vi "Time.vi"(8 "error in (no error)":errorcluster, 10 "Control In":T1={"I-O.lvclass"=refnum, "Gantry"=refnum, "Dispenser"="COM1"}, 11 "Sensor Dispense in":refnum<class "Sensor Dispense.lvclass">) -> (0 "error out":errorcluster, 1 "Timing Data":i32[](array[numeric]), 2 "Control Out":T1={"I-O.lvclass"=refnum, "Gantry"=refnum, "Dispenser"="COM1"}, 3 "Sensor Dispense out":refnum<class "Sensor Dispense.lvclass">)   [LabVIEW 2018, in "Sensor Dispense.lvclass"]
uses:
  Projects/Sensor Dispense.lvclass
  C:/Users/HEP/Documents/GitHub/New folder/C/Users/HEP/Documents/GitHub/UCSB-Gantry-HEP-2018/Classes/Routine/Dispense/Dispense.lvclass
  Controller/Controllers.ctl
  Controller/I-O/I-O.lvclass
  C:/Program Files (x86)/Aerotech/A3200/LabVIEW/2010/Bin/Aerotech.A3200.dll
  Program Files (x86)/Aerotech/A3200/LabVIEW/2010/Bin/Aerotech.A3200.dll
  Projects/Sensor Dispense.lvclass/Sensor Dispense.ctl
  Controller/Motion/Motion.lvclass
  Controller/Motion/A3200/A3200.lvclass
  Controller/Controller.lvclass
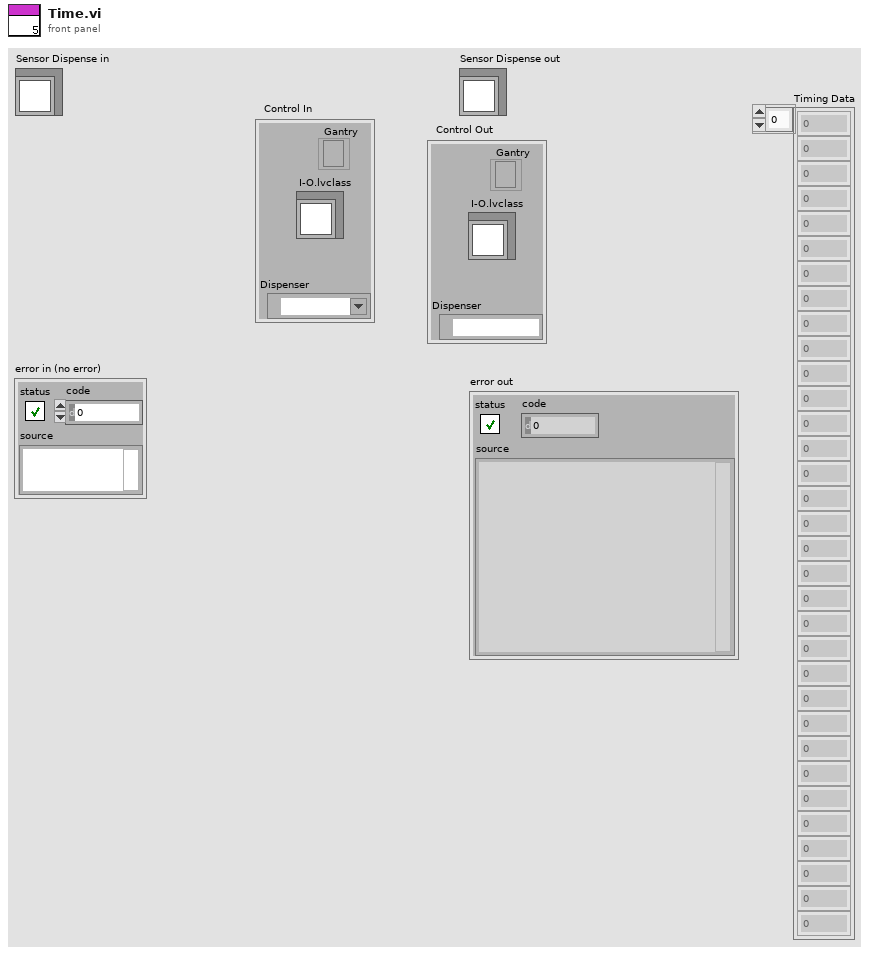
[diagram p1: front panel]
types:
  T1 = typedef "Controller.lvclass/Controllers.ctl" = cluster{"I-O.lvclass":refnum<class "I-O.lvclass">, "Gantry":refnum<k24>, "Dispenser":refnum<visa-resource-name>}
  T2 = cluster{"Endpoints":dbl[][], "Center":dbl[], "CW/CCW":dbl, "Dispense Type":enum16{"N-gon", "Square", "Arc", "Dot", "Line", "Circle"}}[]
  T3 = enum16{"N-gon", "Square", "Arc", "Dot", "Line", "Circle"}
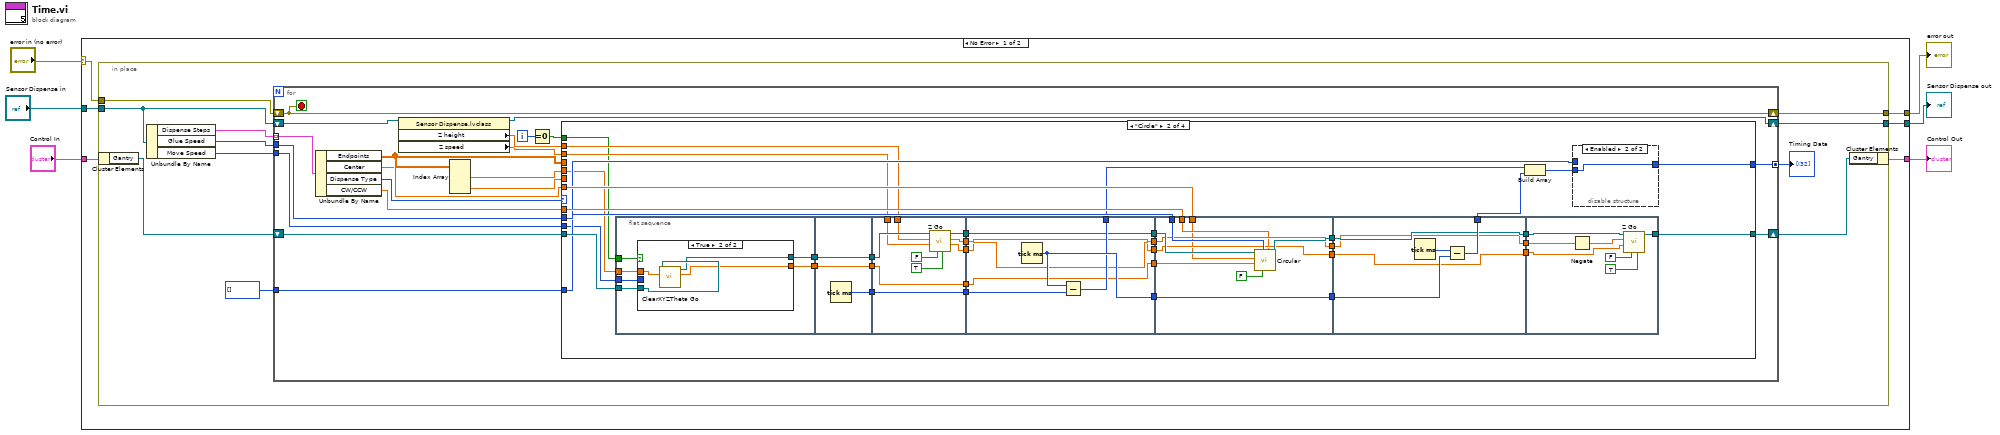
[diagram p0: block diagram]
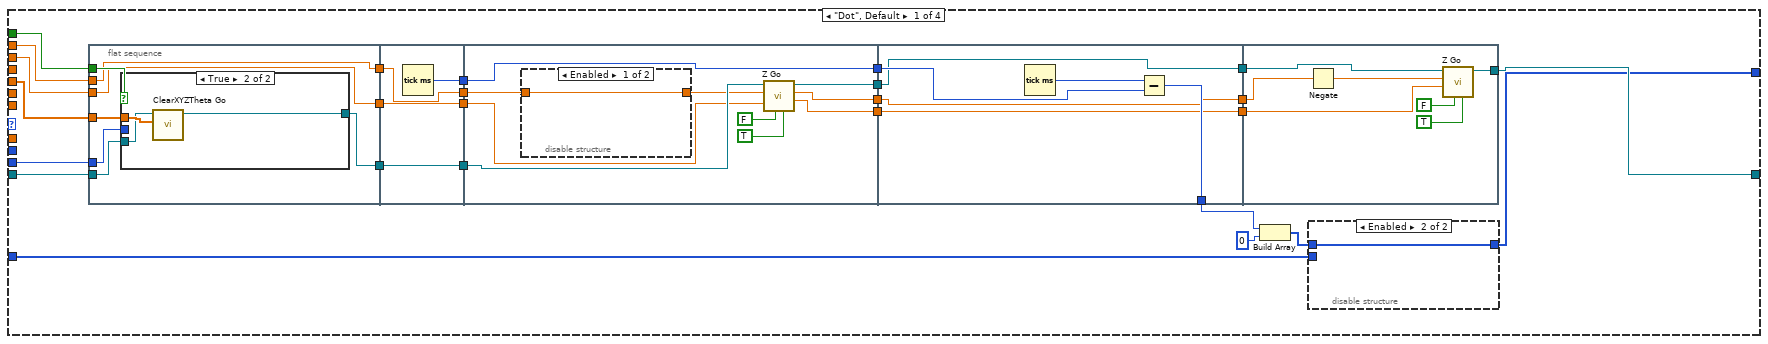
[diagram p2: hidden frame]
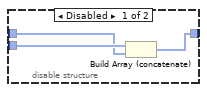
[diagram p3: hidden frame]
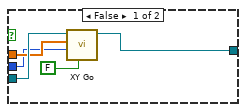
[diagram p4: hidden frame]
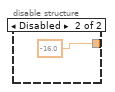
[diagram p5: hidden frame]
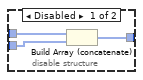
[diagram p6: hidden frame]
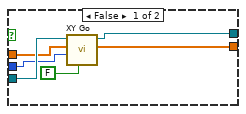
[diagram p7: hidden frame]
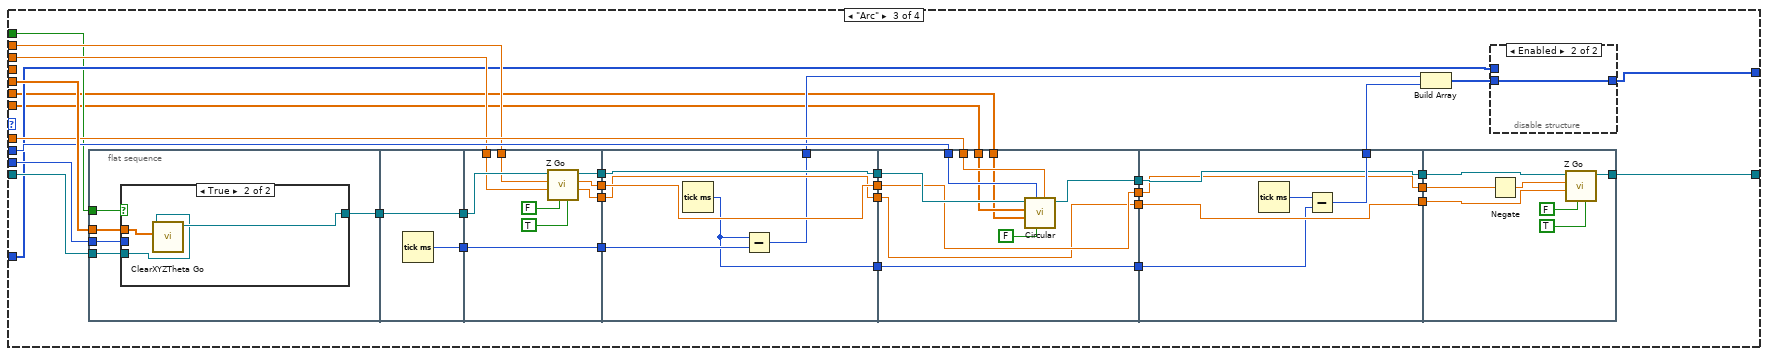
[diagram p8: hidden frame]
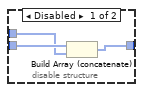
[diagram p9: hidden frame]
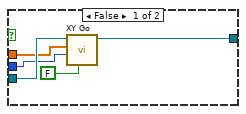
[diagram p10: hidden frame]
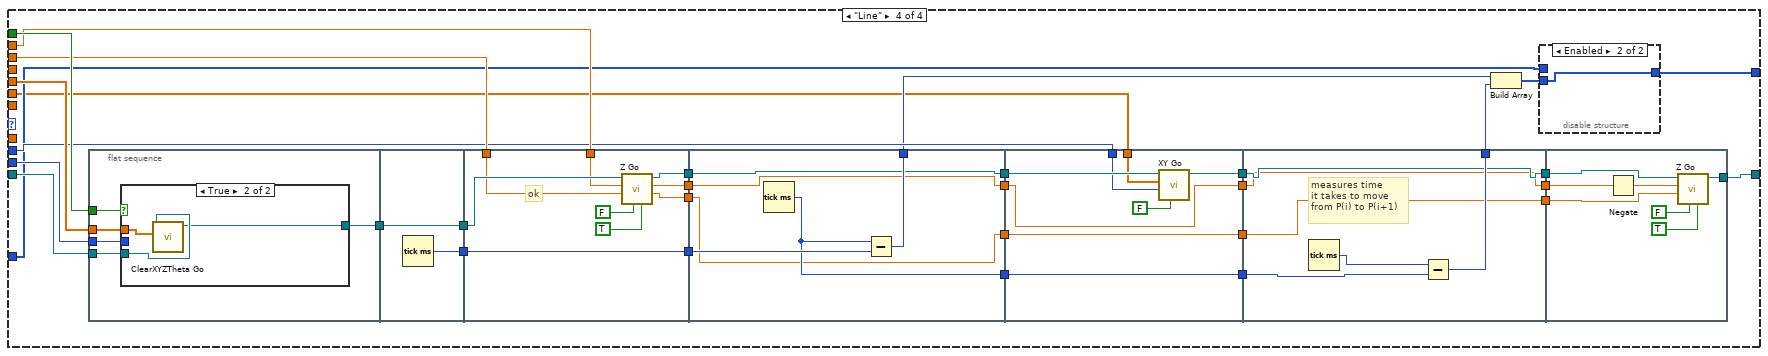
[diagram p11: hidden frame]
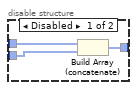
[diagram p12: hidden frame]
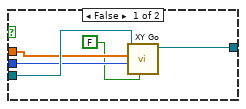
[diagram p13: hidden frame]
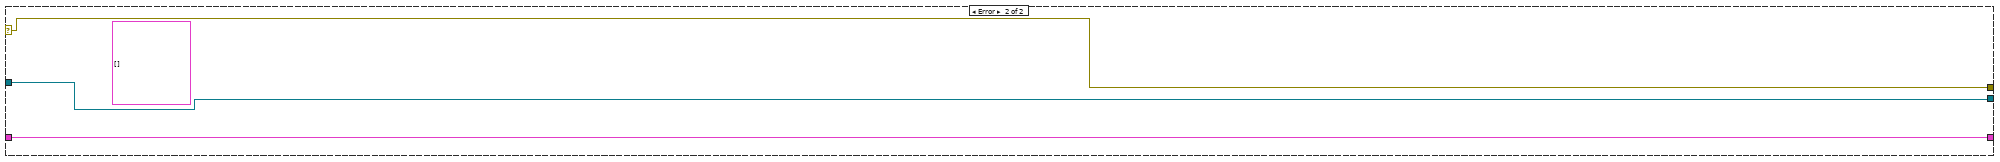
[diagram p14: hidden frame]
diagram:
  n1 = case shown="No Error" "error in (no error)" {
    selector: "error in (no error)" -> [w7 w398]
    tunnel: "Sensor Dispense in" -> [w12 w396]
    tunnel: [w11 w396] -> w5
    tunnel: "Control In" -> [w10 w397]
    tunnel: [w9 w397] -> w3
    tunnel: [w8 w398] -> w2
    frame No Error {
      n2 = in-place {
        in-place-border: w12 -> [w21]
        in-place-border: [w20] -> w11
        in-place-border: [w16] -> w8
        in-place-border: w7 -> [w15]
        n3 = in-place-cluster #1(w10) -> ("Gantry"=w22:refnum<k24>)
        n4 = Unbundle By Name "Unbundle By Name"(w21) -> ("Dispense Steps"=w17:T2, "Glue Speed"=w13:i32, "Move Speed"=w14:i32)
        n5 = for {
          tunnel: w14 -> [w43]
          shift-right: [w30] -> w19
          shift-left: w22 -> [w41]
          tunnel: w13 -> [w26]
          shift-right: [w39] -> w20
          shift-left: w21 -> [w40]
          tunnel: w17 -> [w33] mode=indexing
          shift-right: [w24] -> w16
          shift-left: w15 -> [w24]
          tunnel: i32[] [] -> [w42]
          tunnel: [w34] -> w18 mode=concatenating
          i -> [w38]
          stop <- w24 stop-if-true
          n6 = Unbundle By Name(w33) -> ("Endpoints"=w29:dbl[][], "Center"=w27:dbl[], "Dispense Type"=w32:T3, "CW/CCW"=w25:dbl)
          n7 = property class="Sensor Dispense.lvclass"(reference=w40) -> (reference out=w39:refnum<class "Sensor Dispense.lvclass">, "Z height"=w36:dbl, "Z speed"=w35:dbl)  [unwired: 1 in, 1 out]
          n8 = Index Array(array=w29) -> (element #1=w31:dbl[], element #2=w28:dbl[])  [unwired: 4 in]
          n9 = Equal To 0?(x=w38) -> (x = 0?=w37:bool)
          n10 = case shown="\"Circle\"" w32 {
            tunnel: w27 -> [_ w142 w226 _]
            tunnel: w41 -> [w65 w143 w251 w340]
            tunnel: w43 -> [w49 w131 w249 w338]
            tunnel: [w50 w150 w238 w314] -> w30
            tunnel: w26 -> [_ w141 w248 w328]
            tunnel: w25 -> [_ w140 w247 _]
            tunnel: w42 -> [w46 w137 w230 w312]
            tunnel: [w44 w135 w229 w310] -> w34
            tunnel: w31 -> [w66 w130 w250 w339]
            tunnel: w35 -> [w59 w133 w245 w333]
            tunnel: w36 -> [w62 w134 w246 w334]
            tunnel: w37 -> [w67 w132 w228 w337]
            tunnel: w29 -> [_ _ _ _]
            tunnel: w28 -> [_ _ w227 w309]
            frame "Dot", Default {
              n11 = flat-sequence {
                tunnel: w67 -> [w80]
                tunnel: w66 -> [w79]
                tunnel: w65 -> [w78]
                tunnel: [w77] -> w63
                tunnel: w62 -> [w76]
                tunnel: [w76] -> w60
                tunnel: w59 -> [w75]
                tunnel: [w75] -> w57
                tunnel: w49 -> [w74]
                tunnel: [w92] -> w69
                tunnel: [w91] -> w64
                tunnel: w63 -> [w91]
                tunnel: [w90] -> w61
                tunnel: w60 -> [w90]
                tunnel: [w89] -> w58
                tunnel: w57 -> [w89]
                tunnel: [w102] -> w68
                tunnel: w69 -> [w102]
                tunnel: w64 -> [w101]
                tunnel: w61 -> [w94]
                tunnel: w58 -> [w100]
                tunnel: [w99] -> w55
                tunnel: [w98] -> w53
                tunnel: [w97] -> w51
                tunnel: w68 -> [w110]
                tunnel: [w108] -> w48
                tunnel: [w107] -> w56
                tunnel: w55 -> [w107]
                tunnel: [w106] -> w54
                tunnel: w53 -> [w106]
                tunnel: [w105] -> w52
                tunnel: w51 -> [w105]
                tunnel: w56 -> [w117]
                tunnel: w54 -> [w115]
                tunnel: w52 -> [w114]
                tunnel: [w113] -> w50
                frame #0 {
                  n12 = case shown="True" w80 {
                    tunnel: w79 -> [w83 w88]
                    tunnel: w78 -> [w85 w87]
                    tunnel: [w84 w86] -> w77
                    tunnel: w74 -> [w82 _]
                    frame False {
                      n13 = call "XY Go.vi"("return immediately"=FALSE, "Speed"=w82, "XY In"=w83, "Gantry In"=w85) -> ("Gantry Out"=w84:refnum<k24>)  [unwired: 5 in, 2 out]
                    }
                    frame True {
                      n14 = call "ClearXYZTheta Go.vi"("XYZTheta In"=w88, "Gantry In"=w87) -> ("Gantry Out"=w86:refnum<k24>)  [unwired: 7 in, 2 out]
                    }
                  }
                }
                frame #1 {
                  n15 = Tick Count (ms)() -> (millisecond timer value=w92:u32)
                }
                frame #2 {
                  n16 = disable-structure shown="Enabled" {
                    disable-tunnel: w94 -> [w103 _]
                    disable-tunnel: [w103 -16.0 ("Z height")] -> w93
                    frame Enabled {
                    }
                    frame Disabled {
                    }
                  }
                  n17 = call "Z Go.vi"("Increment"=TRUE, "Return Immediately"=FALSE, "Speed In"=w100, "Position In"=w93, "Gantry In"=w101) -> ("Speed Out"=w98:dbl, "Position Out"=w99:dbl, "Gantry Out"=w97:refnum<k24>)  [unwired: 3 in, 1 out]
                }
                frame #3 {
                  n18 = Tick Count (ms)() -> (millisecond timer value=w109:u32)
                  n19 = Subtract(x=w109, y=w110) -> (x-y=w108:u32)
                }
                frame #4 {
                  n20 = Negate(x=w117) -> (-x=w116:dbl)
                  n21 = call "Z Go.vi"("Increment"=TRUE, "Return Immediately"=FALSE, "Speed In"=w115, "Position In"=w116, "Gantry In"=w114) -> ("Gantry Out"=w113:refnum<k24>)  [unwired: 3 in, 3 out]
                }
              }
              n22 = Build Array(w48, u32 0 ("element")) -> (w45:u32[])
              n23 = disable-structure shown="Enabled" {
                disable-tunnel: w46 -> [w72 _]
                disable-tunnel: w45 -> [w71 w73]
                disable-tunnel: [w70 w73] -> w44
                frame Disabled {
                  n24 = Build Array (concatenate)(w72, w71) -> (w70:u32[])
                }
                frame Enabled {
                }
              }
            }
            frame "Circle" {
              n25 = flat-sequence {
                tunnel: [w161] -> w148
                tunnel: w143 -> [w162]
                tunnel: w130 -> [w163]
                tunnel: w132 -> [w164]
                tunnel: w131 -> [w160]
                tunnel: [w159] -> w126
                tunnel: [w177] -> w154
                tunnel: [w176] -> w149
                tunnel: w148 -> [w176]
                tunnel: [w175] -> w127
                tunnel: w126 -> [w175]
                tunnel: w154 -> [w187]
                tunnel: [w187] -> w153
                tunnel: w149 -> [w185]
                tunnel: [w184] -> w147
                tunnel: w134 -> [w183]
                tunnel: w133 -> [w182]
                tunnel: [w186] -> w128
                tunnel: w127 -> [w186]
                tunnel: [w181] -> w123
                tunnel: [w180] -> w120
                tunnel: w153 -> [w194]
                tunnel: [w193] -> w151
                tunnel: [w192] -> w139
                tunnel: w147 -> [w191]
                tunnel: [w191] -> w146
                tunnel: [w190] -> w129
                tunnel: w128 -> [w190]
                tunnel: [w189] -> w124
                tunnel: w123 -> [w189]
                tunnel: [w188] -> w121
                tunnel: w120 -> [w188]
                tunnel: [w204] -> w152
                tunnel: w151 -> [w204]
                tunnel: w146 -> [w203]
                tunnel: [w202] -> w144
                tunnel: w142 -> [w196]
                tunnel: w141 -> [w201]
                tunnel: w140 -> [w198]
                tunnel: w129 -> [w197]
                tunnel: [w200] -> w125
                tunnel: w124 -> [w200]
                tunnel: [w199] -> w122
                tunnel: w121 -> [w199]
                tunnel: w152 -> [w209]
                tunnel: [w208] -> w138
                tunnel: [w207] -> w145
                tunnel: w144 -> [w207]
                tunnel: w125 -> [w206]
                tunnel: w122 -> [w205]
                tunnel: [w206] -> w119
                tunnel: [w205] -> w118
                tunnel: [w215] -> w150
                tunnel: w145 -> [w216]
                tunnel: w119 -> [w217]
                tunnel: w118 -> [w214]
                frame #0 {
                  n26 = case shown="True" w164 {
                    tunnel: w163 -> [w165 w172]
                    tunnel: w162 -> [w170 w174]
                    tunnel: [w169 w173] -> w161
                    tunnel: w160 -> [w168 _]
                    tunnel: [w167 w171] -> w159
                    frame False {
                      n27 = call "XY Go.vi"("return immediately"=FALSE, "Speed"=w168, "XY In"=w165, "Gantry In"=w170) -> ("XY Out"=w167:dbl[], "Gantry Out"=w169:refnum<k24>)  [unwired: 5 in, 1 out]
                    }
                    frame True {
                      n28 = call "ClearXYZTheta Go.vi"("XYZTheta In"=w172, "Gantry In"=w174) -> ("XYZTheta Out"=w171:dbl[], "Gantry Out"=w173:refnum<k24>)  [unwired: 7 in, 1 out]
                    }
                  }
                }
                frame #1 {
                  n29 = Tick Count (ms)() -> (millisecond timer value=w177:u32)
                }
                frame #2 {
                  n30 = call "Z Go.vi"("Increment"=TRUE, "Return Immediately"=FALSE, "Speed In"=w182, "Position In"=w183, "Gantry In"=w185) -> ("Speed Out"=w180:dbl, "Position Out"=w181:dbl, "Gantry Out"=w184:refnum<k24>)  [unwired: 3 in, 1 out]
                }
                frame #3 {
                  n31 = Tick Count (ms)() -> (millisecond timer value=w193:u32)
                  n32 = Subtract(x=w193, y=w194) -> (x-y=w192:u32)
                }
                frame #4 {
                  n33 = call "Circular.vi"("Direction"=w198, "return immediately"=FALSE, "Speed"=w201, "XY End"=w197, "XY Center"=w196, "Gantry In"=w203) -> ("Gantry Out"=w202:refnum<k24>)  [unwired: 4 in, 1 out]
                }
                frame #5 {
                  n34 = Tick Count (ms)() -> (millisecond timer value=w210:u32)
                  n35 = Subtract(x=w210, y=w209) -> (x-y=w208:u32)
                }
                frame #6 {
                  n36 = Negate(x=w217) -> (-x=w213:dbl)
                  n37 = call "Z Go.vi"("Increment"=TRUE, "Return Immediately"=FALSE, "Speed In"=w214, "Position In"=w213, "Gantry In"=w216) -> ("Gantry Out"=w215:refnum<k24>)  [unwired: 3 in, 3 out]
                }
              }
              n38 = Build Array(w139, w138) -> (w136:u32[])
              n39 = disable-structure shown="Enabled" {
                disable-tunnel: w137 -> [w157 _]
                disable-tunnel: w136 -> [w156 w158]
                disable-tunnel: [w155 w158] -> w135
                frame Disabled {
                  n40 = Build Array (concatenate)(w157, w156) -> (w155:u32[])
                }
                frame Enabled {
                }
              }
            }
            frame "Arc" {
              n41 = flat-sequence {
                tunnel: w251 -> [w260]
                tunnel: w250 -> [w259]
                tunnel: w249 -> [w258]
                tunnel: [w257] -> w242
                tunnel: w228 -> [w256]
                tunnel: w242 -> [w270]
                tunnel: [w270] -> w241
                tunnel: [w269] -> w239
                tunnel: w241 -> [w279]
                tunnel: [w276] -> w244
                tunnel: w246 -> [w278]
                tunnel: w245 -> [w277]
                tunnel: [w275] -> w240
                tunnel: w239 -> [w275]
                tunnel: [w274] -> w236
                tunnel: [w273] -> w234
                tunnel: w244 -> [w285]
                tunnel: [w285] -> w243
                tunnel: w240 -> [w284]
                tunnel: [w283] -> w237
                tunnel: w236 -> [w283]
                tunnel: [w282] -> w235
                tunnel: w234 -> [w282]
                tunnel: [w281] -> w233
                tunnel: [w280] -> w219
                tunnel: w243 -> [w295]
                tunnel: w248 -> [w294]
                tunnel: w247 -> [w293]
                tunnel: w237 -> [w289]
                tunnel: w235 -> [w288]
                tunnel: w226 -> [w292]
                tunnel: w227 -> [w291]
                tunnel: [w290] -> w224
                tunnel: [w289] -> w222
                tunnel: [w288] -> w220
                tunnel: w219 -> [w287]
                tunnel: [w287] -> w218
                tunnel: [w301] -> w232
                tunnel: [w300] -> w225
                tunnel: w224 -> [w300]
                tunnel: [w299] -> w223
                tunnel: w222 -> [w299]
                tunnel: [w298] -> w221
                tunnel: w220 -> [w298]
                tunnel: w218 -> [w296]
                tunnel: [w308] -> w238
                tunnel: w225 -> [w306]
                tunnel: w223 -> [w305]
                tunnel: w221 -> [w304]
                frame #0 {
                  n42 = case shown="True" w256 {
                    tunnel: [w265 w268] -> w257
                    tunnel: w260 -> [w264 w267]
                    tunnel: w259 -> [w261 w266]
                    tunnel: w258 -> [w263 _]
                    frame False {
                      n43 = call "XY Go.vi"("return immediately"=FALSE, "Speed"=w263, "XY In"=w261, "Gantry In"=w264) -> ("Gantry Out"=w265:refnum<k24>)  [unwired: 5 in, 2 out]
                    }
                    frame True {
                      n44 = call "ClearXYZTheta Go.vi"("XYZTheta In"=w266, "Gantry In"=w267) -> ("Gantry Out"=w268:refnum<k24>)  [unwired: 7 in, 2 out]
                    }
                  }
                }
                frame #1 {
                  n45 = Tick Count (ms)() -> (millisecond timer value=w269:u32)
                }
                frame #2 {
                  n46 = call "Z Go.vi"("Increment"=TRUE, "Return Immediately"=FALSE, "Speed In"=w277, "Position In"=w278, "Gantry In"=w279) -> ("Speed Out"=w273:dbl, "Position Out"=w274:dbl, "Gantry Out"=w276:refnum<k24>)  [unwired: 3 in, 1 out]
                }
                frame #3 {
                  n47 = Tick Count (ms)() -> (millisecond timer value=w280:u32)
                  n48 = Subtract(x=w280, y=w284) -> (x-y=w281:u32)
                }
                frame #4 {
                  n49 = call "Circular.vi"("Direction"=w293, "return immediately"=FALSE, "Speed"=w294, "XY End"=w291, "XY Center"=w292, "Gantry In"=w295) -> ("Gantry Out"=w290:refnum<k24>)  [unwired: 4 in, 1 out]
                }
                frame #5 {
                  n50 = Tick Count (ms)() -> (millisecond timer value=w297:u32)
                  n51 = Subtract(x=w297, y=w296) -> (x-y=w301:u32)
                }
                frame #6 {
                  n52 = Negate(x=w305) -> (-x=w307:dbl)
                  n53 = call "Z Go.vi"("Increment"=TRUE, "Return Immediately"=FALSE, "Speed In"=w304, "Position In"=w307, "Gantry In"=w306) -> ("Gantry Out"=w308:refnum<k24>)  [unwired: 3 in, 3 out]
                }
              }
              n54 = Build Array(w233, w232) -> (w231:u32[])
              n55 = disable-structure shown="Enabled" {
                disable-tunnel: w231 -> [w254 w255]
                disable-tunnel: w230 -> [w253 _]
                disable-tunnel: [w252 w255] -> w229
                frame Disabled {
                  n56 = Build Array (concatenate)(w254, w253) -> (w252:u32[])
                }
                frame Enabled {
                }
              }
            }
            frame "Line" {
              n57 = flat-sequence {
                tunnel: w340 -> [w349]
                tunnel: w339 -> [w345]
                tunnel: w338 -> [w348]
                tunnel: w337 -> [w347]
                tunnel: [w346] -> w336
                tunnel: w336 -> [w358]
                tunnel: [w358] -> w335
                tunnel: [w359] -> w331
                tunnel: w335 -> [w368]
                tunnel: w334 -> [w367]
                tunnel: w333 -> [w366]
                tunnel: [w365] -> w332
                tunnel: w331 -> [w365]
                tunnel: [w364] -> w329
                tunnel: [w363] -> w320
                tunnel: [w362] -> w316
                tunnel: w332 -> [w374]
                tunnel: [w373] -> w313
                tunnel: [w372] -> w330
                tunnel: w329 -> [w372]
                tunnel: [w371] -> w326
                tunnel: [w370] -> w321
                tunnel: w320 -> [w370]
                tunnel: [w369] -> w317
                tunnel: w316 -> [w369]
                tunnel: w330 -> [w382]
                tunnel: w328 -> [w381]
                tunnel: [w380] -> w327
                tunnel: w326 -> [w380]
                tunnel: [w379] -> w324
                tunnel: [w378] -> w322
                tunnel: w321 -> [w378]
                tunnel: [w377] -> w318
                tunnel: w317 -> [w377]
                tunnel: w309 -> [w376]
                tunnel: w327 -> [w387]
                tunnel: [w386] -> w315
                tunnel: [w385] -> w325
                tunnel: w324 -> [w385]
                tunnel: [w384] -> w323
                tunnel: w322 -> [w384]
                tunnel: [w383] -> w319
                tunnel: w318 -> [w383]
                tunnel: w325 -> [w395]
                tunnel: w323 -> [w394]
                tunnel: w319 -> [w392]
                tunnel: [w391] -> w314
                frame #0 {
                  n58 = case shown="True" w347 {
                    tunnel: w349 -> [w354 w357]
                    tunnel: w348 -> [w353 _]
                    tunnel: [w352 w356] -> w346
                    tunnel: w345 -> [w351 w355]
                    frame False {
                      n59 = call "XY Go.vi"("return immediately"=FALSE, "Speed"=w353, "XY In"=w351, "Gantry In"=w354) -> ("Gantry Out"=w352:refnum<k24>)  [unwired: 5 in, 2 out]
                    }
                    frame True {
                      n60 = call "ClearXYZTheta Go.vi"("XYZTheta In"=w355, "Gantry In"=w357) -> ("Gantry Out"=w356:refnum<k24>)  [unwired: 7 in, 2 out]
                    }
                  }
                }
                frame #1 {
                  n61 = Tick Count (ms)() -> (millisecond timer value=w359:u32)
                }
                frame #2 {
                  # "ok"
                  n62 = call "Z Go.vi"("Increment"=TRUE, "Return Immediately"=FALSE, "Speed In"=w366, "Position In"=w367, "Gantry In"=w368) -> ("Speed Out"=w362:dbl, "Position Out"=w363:dbl, "Gantry Out"=w364:refnum<k24>)  [unwired: 3 in, 1 out]
                }
                frame #3 {
                  n63 = Tick Count (ms)() -> (millisecond timer value=w371:u32)
                  n64 = Subtract(x=w371, y=w374) -> (x-y=w373:u32)
                }
                frame #4 {
                  n65 = call "XY Go.vi"("return immediately"=FALSE, "Speed"=w381, "XY In"=w376, "Gantry In"=w382) -> ("Gantry Out"=w379:refnum<k24>)  [unwired: 5 in, 2 out]
                }
                frame #5 {
                  # "measures time\nit takes to move\nfrom P(i) to P(i+1)"
                  n66 = Tick Count (ms)() -> (millisecond timer value=w388:u32)
                  n67 = Subtract(x=w388, y=w387) -> (x-y=w386:u32)
                }
                frame #6 {
                  n68 = Negate(x=w394) -> (-x=w393:dbl)
                  n69 = call "Z Go.vi"("Increment"=TRUE, "Return Immediately"=FALSE, "Speed In"=w392, "Position In"=w393, "Gantry In"=w395) -> ("Gantry Out"=w391:refnum<k24>)  [unwired: 3 in, 3 out]
                }
              }
              n70 = Build Array(w313, w315) -> (w311:u32[])
              n71 = disable-structure shown="Enabled" {
                disable-tunnel: w312 -> [w343 _]
                disable-tunnel: w311 -> [w342 w344]
                disable-tunnel: [w341 w344] -> w310
                frame Disabled {
                  n72 = Build Array (concatenate)(w343, w342) -> (w341:u32[])
                }
                frame Enabled {
                }
              }
            }
          }
        }
        "Timing Data" <- w18
        n73 = in-place-cluster #1("Gantry"=w19) -> (w9:T1)
      }
    }
    frame Error {
      (unwired) T2 [] ("Dispense Steps")
    }
  }
  "error out" <- w2
  "Sensor Dispense out" <- w5
  "Control Out" <- w3
